vi "arrays.vi"() -> ()   [LabVIEW 2023]
uses:
  e26876a3-6bbf-4add-a93c-2404d599011b.vi
  <vilib>/Array/Sort 2D Array - Pop Stack.vi
  <vilib>/Array/Sort 2D Array - Push Stack.vi
  e26876a3-6bbf-4add-a93c-2404d599011b.vi/269d4b3b-47f5-49e3-8884-44851e4dd9d5.vi
  e26876a3-6bbf-4add-a93c-2404d599011b.vi/6d99389c-673d-4efb-bf33-19b32bcf4cf8.vi
panel:
  out "Boolean":bool
  out "max val * 10 graph":dbl[](graph)
  out "max val graph":dbl[](graph)
  out "Waveform Chart":dbl(graph)
  in  "wait":u32
  in  "stop":bool
  out "Sorted columns":dbl[][](array[numeric]) format="%#.2g"
  out "Sorted rows":dbl[][](array[numeric]) format="%#.2g"
  out "Array":dbl[][](array[numeric])
  out "Last value":dbl
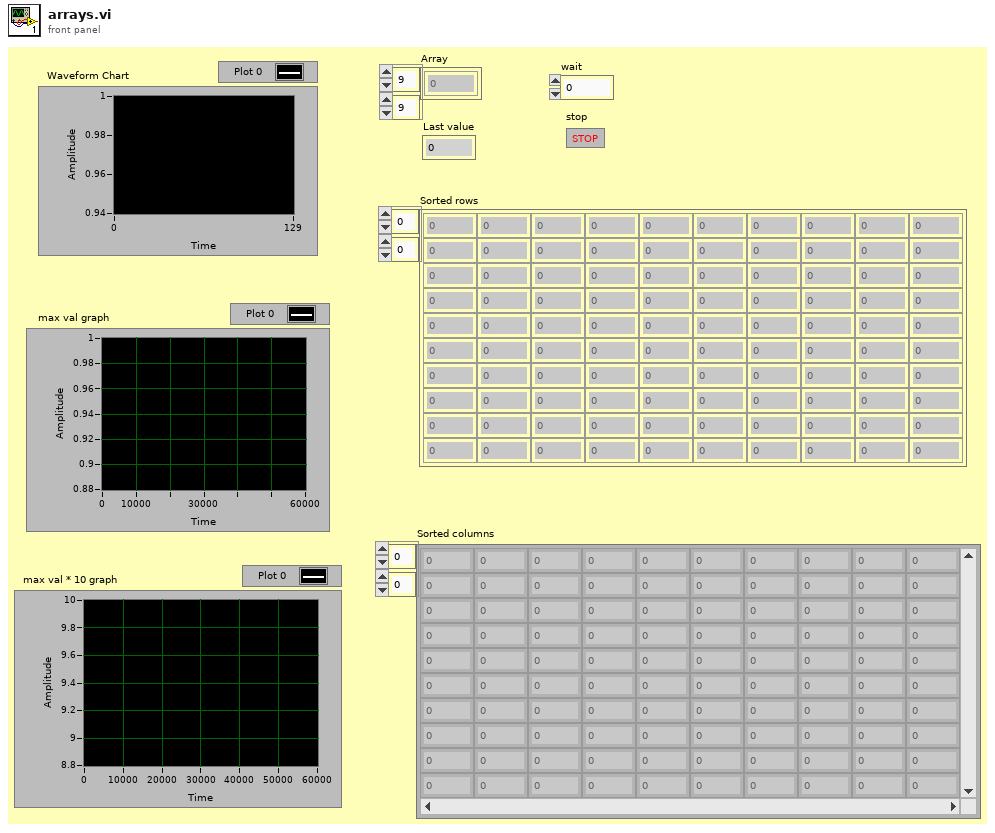
[diagram p1: front panel]
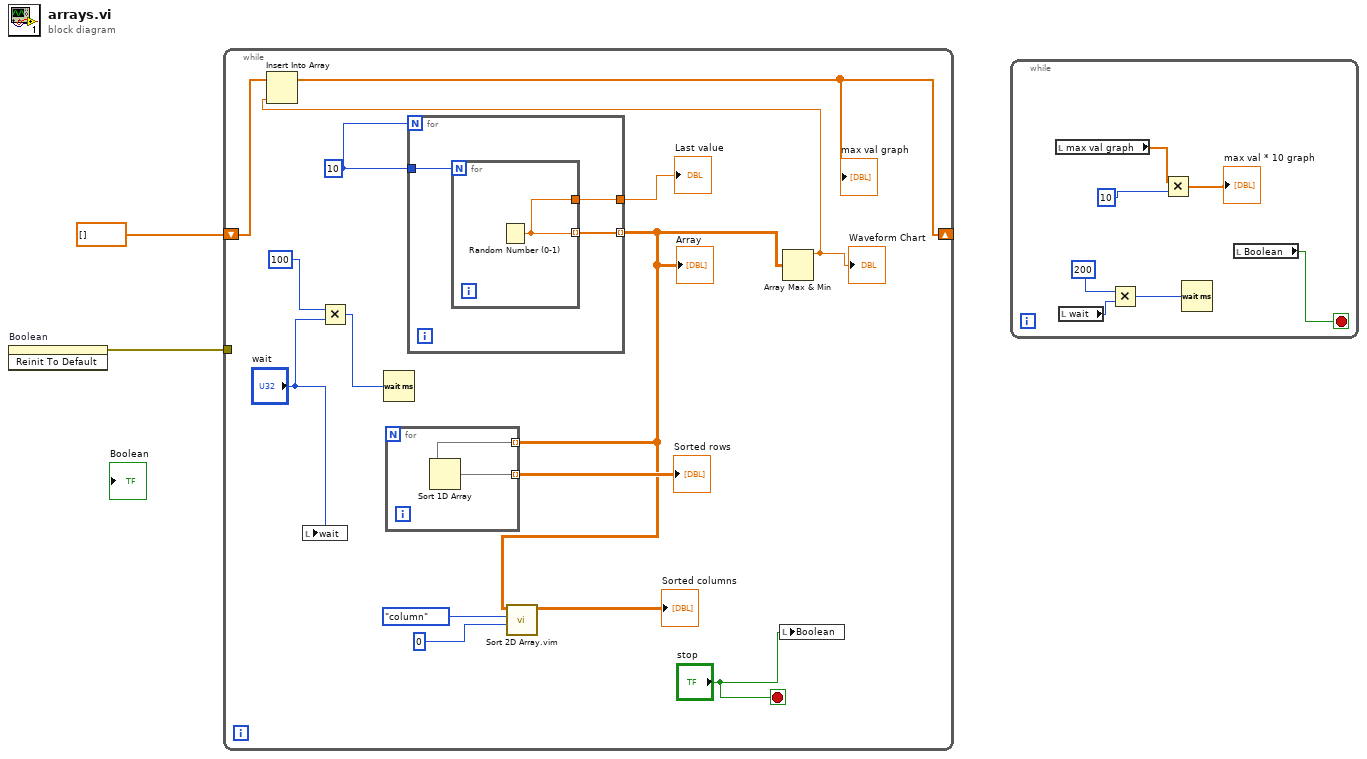
[diagram p0: block diagram]
diagram:
  n1 = invoke on="Boolean" class="Bool (strict)" method="Reinit To Default"() -> (error out=w1:errorcluster)  [unwired: 3 in, 2 out]
  n2 = while {
    shift-right: [w6] -> _
    shift-left: dbl[] [] -> [w8]
    tunnel: w1 -> [_]
    stop <- "stop" stop-if-true
    w11 = 10
    n3 = local write "wait"("wait") -> ()
    n4 = Multiply(x=100, y="wait") -> (x*y=w4:u32)
    n5 = Wait (ms)(milliseconds to wait=w4) -> ()  [unwired: 1 out]
    n6 = for {
      N: w11 -> [_]
      tunnel: w11 -> [w21]
      tunnel: [w19] -> w9 mode=indexing
      tunnel: [w20] -> w16
      n7 = for {
        N: w21 -> [_]
        tunnel: [w22] -> w19 mode=indexing
        tunnel: [w22] -> w20
        n8 = Random Number (0-1)() -> (number: 0 to 1=w22:dbl)
      }
    }
    "Last value" <- w16
    "Array" <- w9
    n9 = for {
      tunnel: w9 -> [w18] mode=indexing
      tunnel: [w17] -> w15 mode=indexing
      n10 = Sort 1D Array(array=w18) -> (sorted array=w17:dbl[])
    }
    "Sorted rows" <- w15
    n11 = call "Sort 2D Array.vim"("index"=0, "dimension to index (column)"=enum16{"column", "row"}."column", "2D array"=w9) -> ("sorted 2D array"=→"Sorted columns":dbl[][])  [unwired: 7 in, 1 out]
    n12 = local write "Boolean"("stop") -> ()
    n13 = Array Max & Min(array=w9) -> (max value=w7:dbl)  [unwired: 3 out]
    "Waveform Chart" <- w7
    n14 = Insert Into Array(array=w8, new element=w7) -> (w6:dbl[])  [unwired: 1 in]
    "max val graph" <- w6
  }
  n15 = while {
    stop <- w24 stop-if-true
    n16 = local read "max val graph"() -> (w28:dbl[])
    n17 = local read "wait"() -> (w23:u32)
    n18 = Multiply(x=200, y=w23) -> (x*y=w25:u32)
    n19 = Multiply(x=w28, y=10) -> (x*y=→"max val * 10 graph":dbl[])
    n20 = Wait (ms)(milliseconds to wait=w25) -> ()  [unwired: 1 out]
    n21 = local read "Boolean"() -> (w24:bool)
  }
